vi "White_Convolve.vi"(5 "# harmonics":i32=40, 7 "signal type":T1(ring), 9 "frequency":dbl=10.0 format="%#_13g", 11 "Complex FRF":cluster{dbl, "df":dbl, cdb[]}) -> (3 "convolution":cluster{dbl, "df":dbl, dbl[]}(graph))   [LabVIEW 2022 SP3]
uses:
  <vilib>/Analysis/4window.llb/Hanning Window (DBL).vi
  <vilib>/Analysis/2dsp.llb/Real FFT.vi
  <vilib>/Analysis/4window.llb/AllCosWindow (DBL).vi
  <vilib>/measure/NI_MABase.lvlib
  <vilib>/Analysis/NI_AALPro.lvlib
panel:
  out "FFT(saw)":cluster{dbl, "df":dbl, dbl[]}(graph)
  out "Comparison":dbl[][](graph)
  out "signal":cluster{dbl, "df":dbl, dbl[]}(graph)
  out "magnitude":cluster{dbl, "df":dbl, dbl[]}(graph)
  out "Waveform":waveform(dbl)(graph)
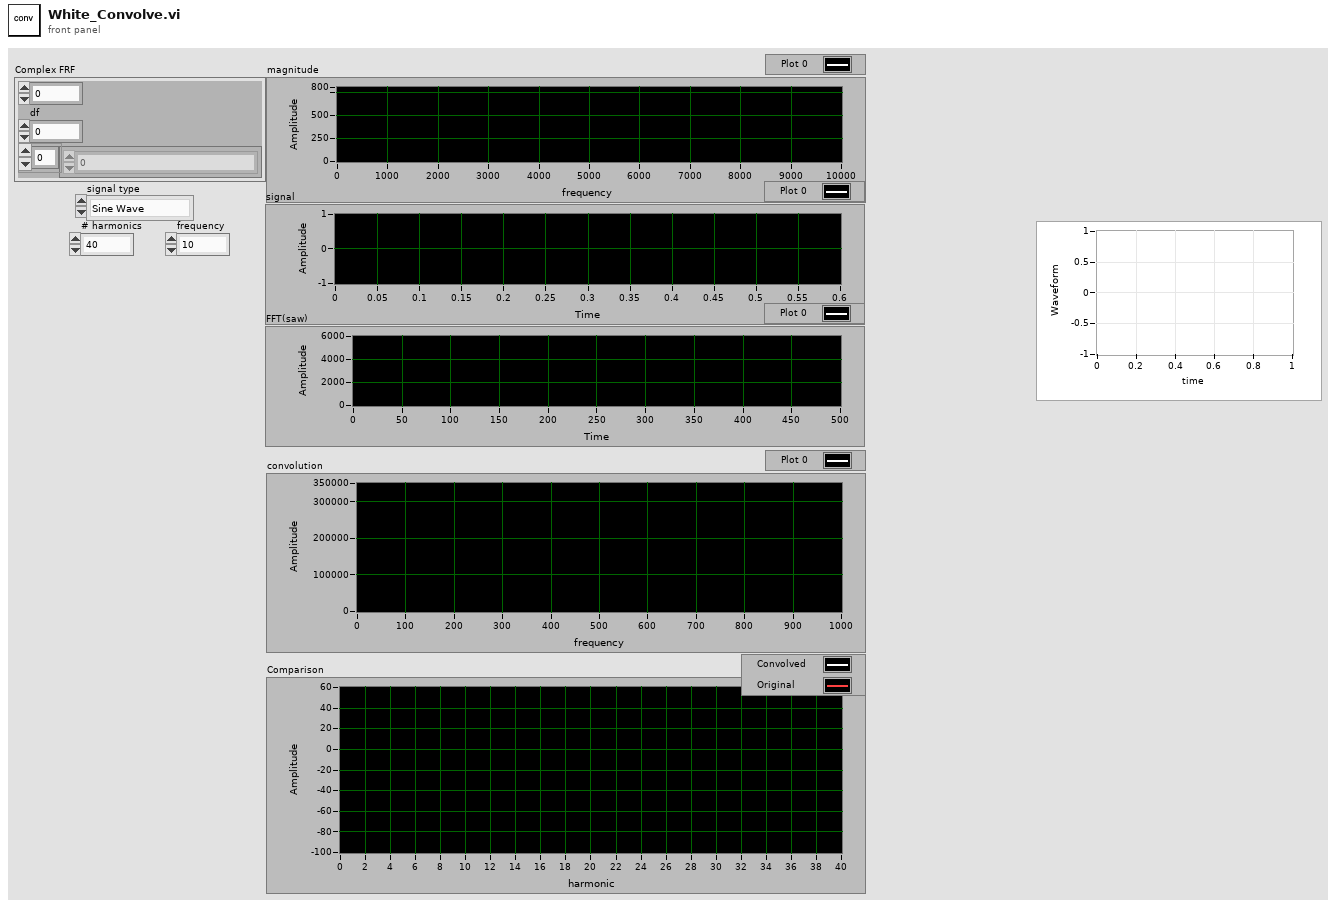
[diagram p1: front panel]
types:
  T1 = enum16{"Sine Wave", "Triangle Wave", "Square Wave", "Sawtooth Wave"}
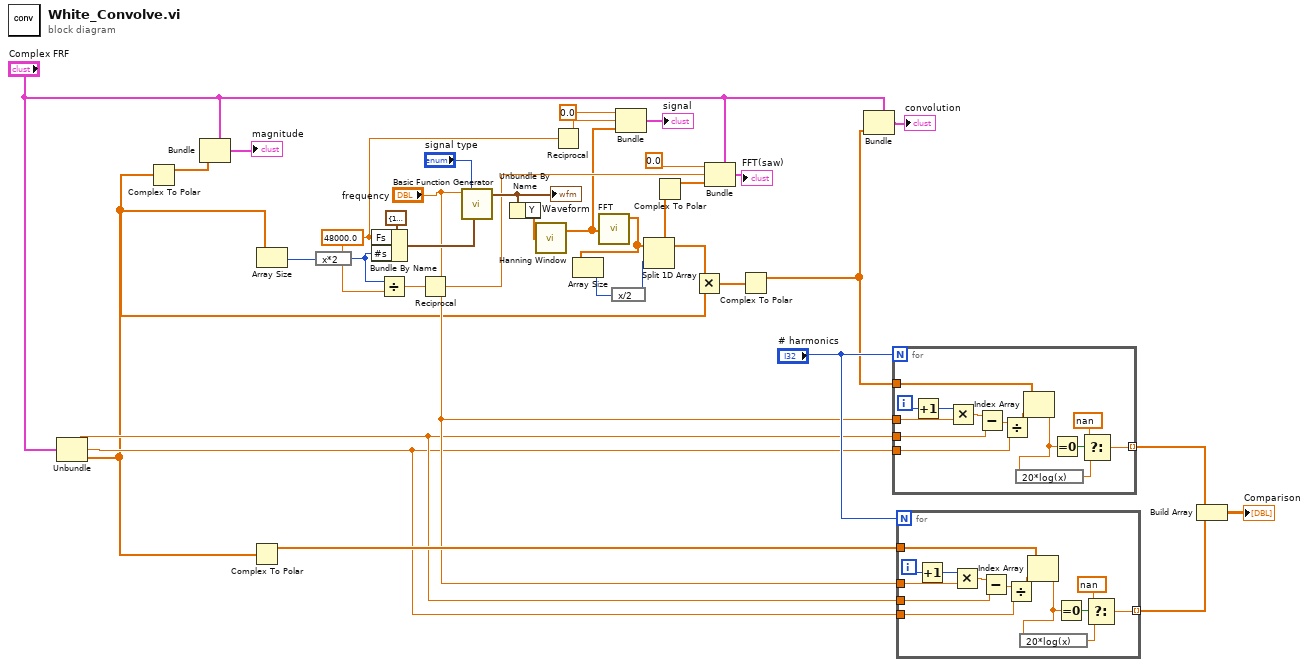
[diagram p0: block diagram]
diagram:
  w2 = 48000.0 ("Fs")
  n1 = Unbundle("Complex FRF") -> (w21:dbl, "df"=w20:dbl, w19:cdb[])
  n2 = Complex To Polar(r * e^(i*theta)=w19) -> (r=w13:dbl[])  [unwired: 1 out]
  n3 = Bundle(cluster="Complex FRF", w13) -> (→"magnitude":cluster{dbl, "df":dbl, cdb[]})  [unwired: 2 in]
  n4 = Complex To Polar(r * e^(i*theta)=w19) -> (r=w28:dbl[])  [unwired: 1 out]
  n5 = Array Size(array=w19) -> (size(s)=w31:i32)
  n6 = expression code="x*2"(w31) -> (w3:i32)
  n7 = Bundle By Name(cluster=cluster{"Fs":dbl, "#s":dbl} {"Fs"=1000.0, "#s"=1000.0} ("sampling info"), "Fs"=w2, "#s"=w3) -> (w35:cluster{"Fs":dbl, "#s":dbl})
  n8 = Divide(x=w3, y=w2) -> (x/y=w7:dbl)
  n9 = Reciprocal(x=w7) -> (1/x=w6:dbl)
  n10 = call <vilib>:"Basic Function Generator.vi"("sampling info"=w35, "signal type"="signal type", "frequency"="frequency") -> ("signal out"=w33:waveform(dbl))  [unwired: 6 in, 2 out]
  "Waveform" <- w33
  n11 = Unbundle By Name(w33) -> ("Y"=w9:dbl[])
  n12 = call-poly <vilib>:"Hanning Window.vi"("X"=w9) -> ("Windowed X"=w1:dbl[])  [unwired: 1 out]
  n13 = Reciprocal(x=w2) -> (1/x=w15:dbl)
  n14 = call-poly <vilib>:"FFT.vi"("X"=w1) -> ("FFT {X}"=w18:cdb[])  [unwired: 9 in, 1 out]
  n15 = Array Size(array=w18) -> (size(s)=w17:i32)
  n16 = expression code="x/2"(w17) -> (w30:i32)
  n17 = Bundle("Fs"=0.0, w15, "Windowed X"=w1) -> (→"signal":cluster{"Fs":dbl, dbl, "Windowed X":dbl[]})  [unwired: 1 in]
  n18 = Split 1D Array(array=w18, index=w30) -> (first subarray=w5:cdb[])  [unwired: 1 out]
  n19 = Complex To Polar(r * e^(i*theta)=w5) -> (r=w4:dbl[])  [unwired: 1 out]
  n20 = Multiply(x=w5, y=w19) -> (x*y=w32:cdb[])
  n21 = Bundle(cluster="Complex FRF", 0.0 ("Fs"), "df"=w6, w4) -> (→"FFT(saw)":cluster{dbl, "df":dbl, cdb[]})
  n22 = Complex To Polar(r * e^(i*theta)=w32) -> (r=w16:dbl[])  [unwired: 1 out]
  n23 = Bundle(cluster="Complex FRF", w16) -> (→"convolution":cluster{dbl, "df":dbl, cdb[]})  [unwired: 2 in]
  n24 = for {
    N: "# harmonics" -> [_]
    tunnel: w16 -> [w50]
    tunnel: "frequency" -> [w46]
    tunnel: w21 -> [w45]
    tunnel: w20 -> [w44]
    tunnel: [w40] -> w23 mode=indexing
    i -> [w42]
    n25 = Increment(x=w42) -> (x+1=w49:i32)
    n26 = Multiply(x=w49, y=w46) -> (x*y=w48:dbl)
    n27 = Subtract(x=w48, y=w45) -> (x-y=w47:dbl)
    n28 = Divide(x=w47, y=w44) -> (x/y=w43:dbl)
    n29 = Index Array(array=w50, index=w43) -> (element=w38:dbl)
    n30 = expression code="20*log(x)"(w38) -> (w37:dbl)
    n31 = Equal To 0?(x=w38) -> (x = 0?=w41:bool)
    n32 = Select(t=nan, s=w41, f=w37) -> (s? t:f=w40:dbl)
  }
  n33 = for {
    N: "# harmonics" -> [_]
    tunnel: w28 -> [w64]
    tunnel: "frequency" -> [w60]
    tunnel: w21 -> [w59]
    tunnel: w20 -> [w58]
    tunnel: [w54] -> w22 mode=indexing
    i -> [w56]
    n34 = Increment(x=w56) -> (x+1=w63:i32)
    n35 = Multiply(x=w63, y=w60) -> (x*y=w62:dbl)
    n36 = Subtract(x=w62, y=w59) -> (x-y=w61:dbl)
    n37 = Divide(x=w61, y=w58) -> (x/y=w57:dbl)
    n38 = Index Array(array=w64, index=w57) -> (element=w52:dbl)
    n39 = expression code="20*log(x)"(w52) -> (w51:dbl)
    n40 = Equal To 0?(x=w52) -> (x = 0?=w55:bool)
    n41 = Select(t=nan, s=w55, f=w51) -> (s? t:f=w54:dbl)
  }
  n42 = Build Array(w23, w22) -> (→"Comparison":dbl[][])
